vi "Write ParameterValues.vi"(8 "error in (no error)":errorcluster, 10 "ParameterValues":variant[](array[variant]), 11 "DynamicParameters in":refnum<class "DynamicParameters.lvclass">) -> (0 "error out":errorcluster, 3 "DynamicParameters out":refnum<class "DynamicParameters.lvclass">)   [LabVIEW 2020, in "ORM.lvlib" / "DynamicParameters.lvclass"]
uses:
  DynamicParameters.lvclass
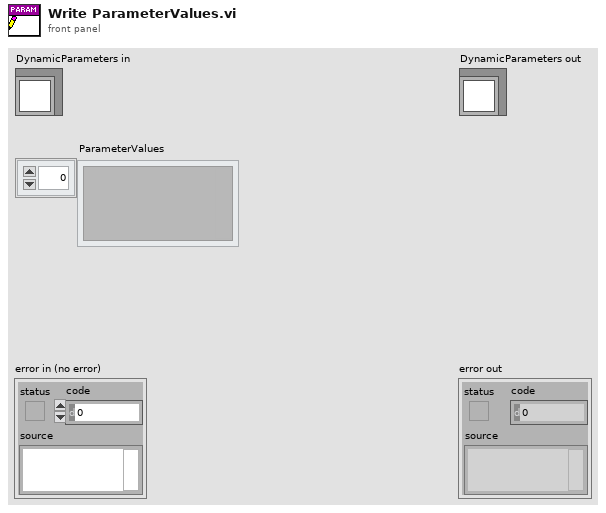
[diagram p1: front panel]
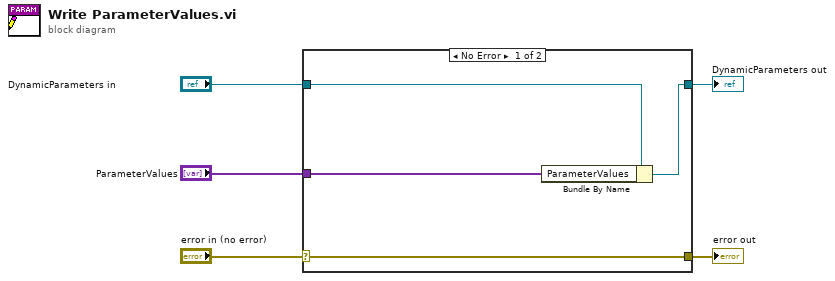
[diagram p0: block diagram]
diagram:
  n1 = case shown="No Error" "error in (no error)" {
    selector: "error in (no error)" -> [w9 w10]
    tunnel: [w9 w10] -> w4
    tunnel: [w7 w11] -> w2
    tunnel: "DynamicParameters in" -> [w8 w11]
    tunnel: "ParameterValues" -> [w6 _]
    frame No Error {
      n2 = Bundle By Name(cluster=w8, "ParameterValues"=w6) -> (w7:refnum<class "DynamicParameters.lvclass">)
    }
    frame Error {
    }
  }
  "error out" <- w4
  "DynamicParameters out" <- w2
